vi "SRV_Get Random Number in Range.vi"(5 "Low (0)":dbl format="%.2f", 7 "Integers only? (F)":bool, 9 "High (10)":dbl=10.0 format="%.2f") -> (8 "Random Number":dbl format="%.2f")   [LabVIEW 2009]
doc: "Gets a random number within the range of the Low/High number values given, inclusively.\n\nIf \"Integers only?\" is TRUE, the floating point result will be rounded to the nearest integer.\n\n\nAuthor: Mike Schultz"
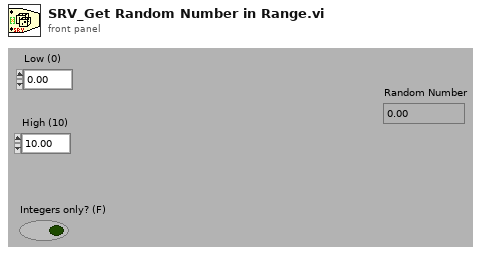
[diagram p1: front panel]
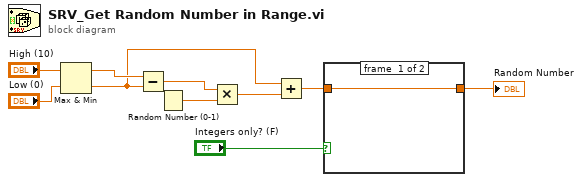
[diagram p0: block diagram]
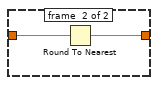
[diagram p2: hidden frame]
diagram:
  n1 = Max & Min(x="High (10)", y="Low (0)") -> (max(x,y)=w4:dbl, min(x,y)=w3:dbl)
  n2 = Subtract(x=w4, y=w3) -> (x-y=w7:dbl)
  n3 = Random Number (0-1)() -> (number: 0 to 1=w8:dbl)
  n4 = Multiply(x=w7, y=w8) -> (x*y=w6:dbl)
  n5 = Add(x=w3, y=w6) -> (x+y=w5:dbl)
  n6 = case shown="True" "Integers only? (F)" {
    tunnel: w5 -> [w11 w13]
    tunnel: [w11 w12] -> w9
    frame #0 {
    }
    frame #1 {
      n7 = Round To Nearest(number=w13) -> (nearest integer value=w12:dbl)
    }
  }
  "Random Number" <- w9
